vi "PythonDebug.vi"(8 "error in (no error)":errorcluster, 10 "img in":T1, 11 "session in":refnum<k35>) -> (0 "error out":errorcluster, 2 "debug string":string, 3 "session out":refnum<k35>)   [LabVIEW 2018]
uses:
  <vilib>/picture/picture.llb/imagedata.ctl
panel:
  # "YOU MAY EDIT THE \"debug()\" FUNTION\nTO RETURN A STRING FOR USE WITH\nDEBUGGING"
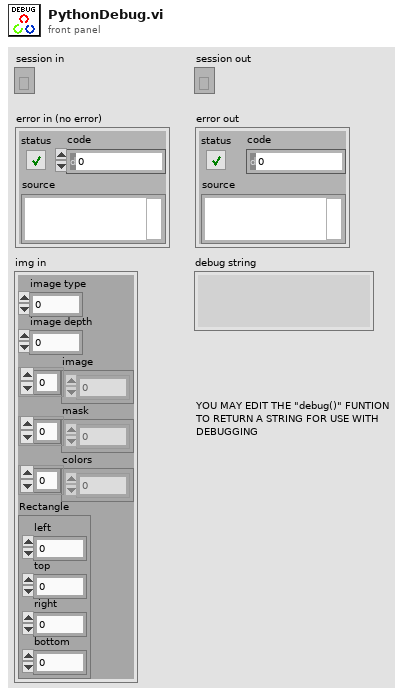
[diagram p1: front panel]
types:
  T1 = typedef "imagedata.ctl" = cluster{"image type":i32, "image depth":i32, "image":u8[], "mask":u8[], "colors":u32[], "Rectangle":cluster{"left":i16, "top":i16, "right":i16, "bottom":i16}}
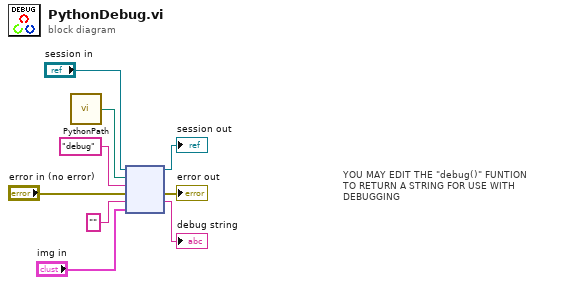
[diagram p0: block diagram]
diagram:
  # "YOU MAY EDIT THE \"debug()\" FUNTION\nTO RETURN A STRING FOR USE WITH\nDEBUGGING"
  n1 = call "PythonPath.vi"() -> ("path to .py"=w4:path)
  n2 = node("session in", w4, "debug" ("function name"), "error in (no error)", "", "img in") -> (→"session out":refnum<k35>, →"error out":errorcluster, →"debug string":string)  [unwired: 1 in, 2 out]
